vi "Position to Key.vi"(4 "Rel Center":u16, 6 "L/R":bool, 8 "Pos y":u16=40, 9 "Pos x":u16=40) -> (1 "Key":u8)   [LabVIEW 2015]
uses:
  TypeDefs Host/Open Audio FGV Enum.ctl
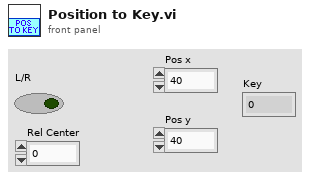
[diagram p1: front panel]
types:
  T1 = typedef "Open Audio FGV Enum.ctl" = enum16{"Get", "Set"}
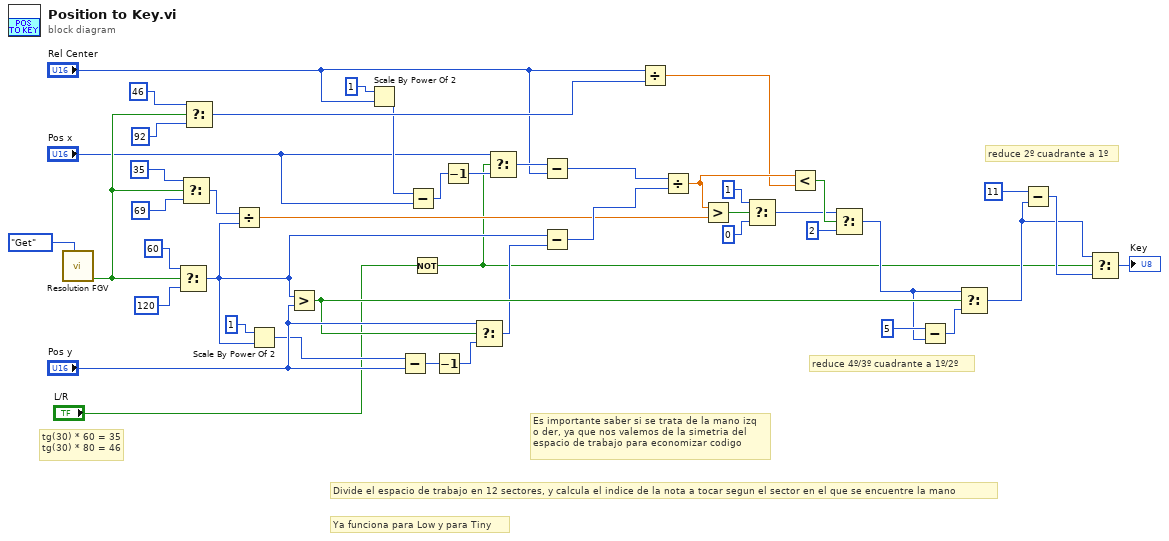
[diagram p0: block diagram]
diagram:
  # "tg(30) * 60 = 35\ntg(30) * 80 = 46"
  # "reduce 2º cuadrante a 1º"
  # "reduce 4º/3º cuadrante a 1º/2º"
  # "Ya funciona para Low y para Tiny"
  # "Es importante saber si se trata de la mano izq\no der, ya que nos valemos de la simetria del \nespacio de trabajo para economizar codigo"
  # "Divide el espacio de trabajo en 12 sectores, y calcula el indice de la nota a tocar segun el sector en el que se encuentre la mano"
  n1 = call "Resolution FGV.vi"("Command"=Open_Audio_FGV_Enum."Get") -> ("L/T?"=w10:bool)  [unwired: 10 in]
  n2 = Select(t=u16 60 ("y"), s=w10, f=u16 120 ("y")) -> (s? t:f=w16:u16)
  n3 = Select(t=u16 35 ("x"), s=w10, f=u16 69 ("x")) -> (s? t:f=w12:u16)
  n4 = Select(t=u16 46 ("y"), s=w10, f=u16 92 ("y")) -> (s? t:f=w7:u16)
  n5 = Divide(x=w12, y=w16) -> (x/y=w15:dbl)
  n6 = Scale By Power Of 2(n=i16 1, x=w16) -> (x*2^n=w17:u16)
  n7 = Greater?(x=w16, y="Pos y") -> (0:w38:bool)
  n8 = Scale By Power Of 2(n=i16 1, x="Rel Center") -> (x*2^n=w6:u16)
  n9 = Subtract(x=w17, y="Pos y") -> (x-y=w40:u16)
  n10 = Subtract(x=w6, y="Pos x") -> (x-y=w33:u16)
  n11 = Not(x="L/R") -> (.not. x?=w1:bool)
  n12 = Decrement(x=w40) -> (x-1=w39:u16)
  n13 = Decrement(x=w33) -> (x-1=w32:u16)
  n14 = Select(t="Pos y", s=w38, f=w39) -> (s? t:f=w30:u16)
  n15 = Select(t="Pos x", s=w1, f=w32) -> (s? t:f=w42:u16)
  n16 = Subtract(x=w42, y="Rel Center") -> (x-y=w31:u16)
  n17 = Subtract(x=w16, y=w30) -> (x-y=w29:u16)
  n18 = Divide(x="Rel Center", y=w7) -> (x/y=w14:dbl)
  n19 = Divide(x=w31, y=w29) -> (x/y=w25:dbl)
  n20 = Greater?(x=w25, y=w15) -> (0:w28:bool)
  n21 = Select(t=u8 1 ("y"), s=w28, f=u8 0 ("y")) -> (s? t:f=w23:u8)
  n22 = Less?(x=w25, y=w14) -> (x < y?=w24:bool)
  n23 = Select(t=w23, s=w24, f=u8 2) -> (s? t:f=w35:u8)
  n24 = Subtract(x=u8 5 ("y"), y=w35) -> (x-y=w34:u8)
  n25 = Select(t=w35, s=w38, f=w34) -> (s? t:f=w37:u8)
  n26 = Subtract(x=u8 11 ("y"), y=w37) -> (x-y=w45:u8)
  n27 = Select(t=w37, s=w1, f=w45) -> (s? t:f=→"Key":u8)
